vi "test Path Functions.vi"(8 "error in (no error)":errorcluster, 11 "TestCase in":refnum<class "Variant Data Manipulation Tests.lvclass">) -> (0 "error out":errorcluster, 3 "TestCase out":refnum<class "Variant Data Manipulation Tests.lvclass">)   [LabVIEW 2017, in "Variant Data Manipulation Tests.lvclass"]
uses:
  Variant Data Manipulation Tests.lvclass
  Source/Path API/Read Value at Path(String).vi
  Source/Path API/Write Value at Path(String).vi
  Source/Path API/Write Label at Path(String).vi
  <vilib>/addons/_JKI Toolkits/VI Tester/TestCase.llb/TestCase.lvclass
  Source/Variant Data Manipulation.lvlib
  C:/Program Files (x86)/National Instruments/LabVIEW 2017/vi.lib/addons/_JKI Toolkits/VI Tester/TestCase.llb/TestCase.lvclass
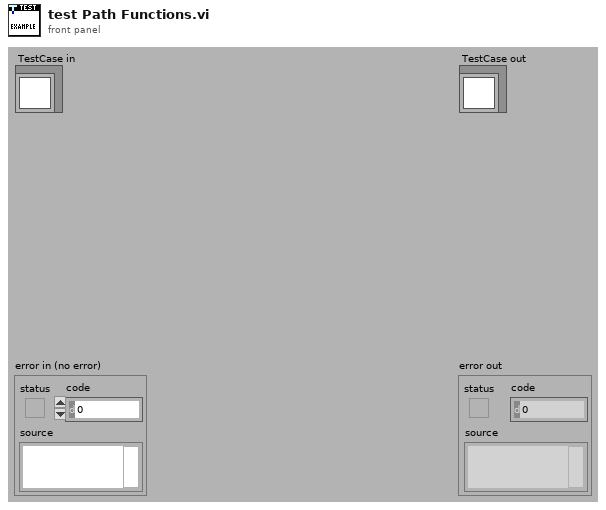
[diagram p1: front panel]
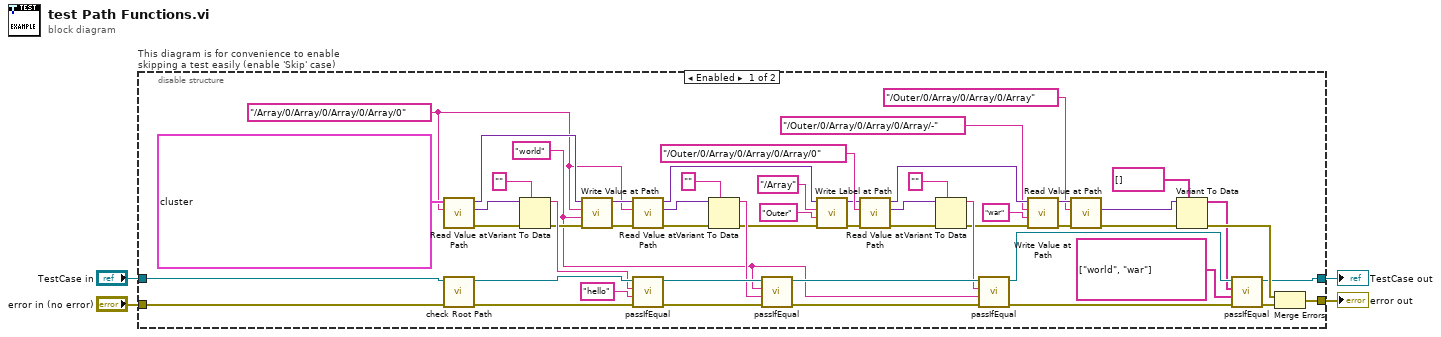
[diagram p0: block diagram]
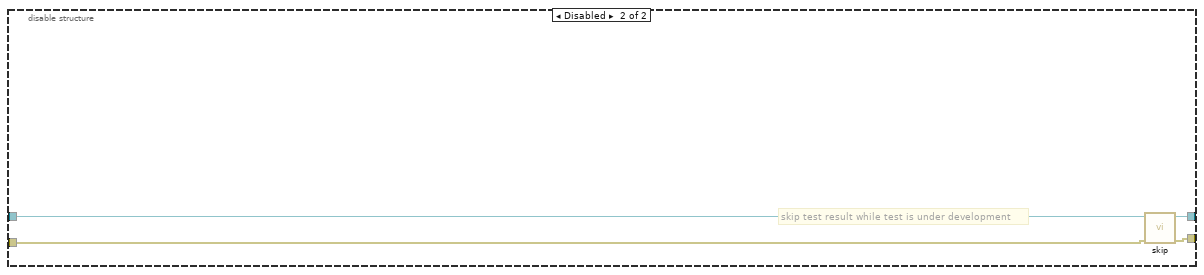
[diagram p2: hidden frame]
diagram:
  n1 = disable-structure "This diagram is for convenience to enable skipping a test easily (enable 'Skip' case)" shown="Enabled" {
    disable-tunnel: "TestCase in" -> [w57 w61]
    disable-tunnel: [w9 w59] -> w1
    disable-tunnel: [w24 w60] -> w3
    disable-tunnel: "error in (no error)" -> [w56 w58]
    frame Enabled {
      w21 = "world" ("String")
      w26 = "/Array/0/Array/0/Array/0/Array/0" ("Path String")
      n2 = call-poly "Read Value at Path.vi"("Path String"=w26, "Variant in"=cluster{"Array":cluster{"Array":cluster[]}[]} {"Array"=[{"Array"=[{"Array"=[{"Array"=["hello"]}]}]}]} ("Cluster")) -> ("error out"=w53:errorcluster, "Element out"=w52:variant, "Variant out"=w46:variant)  [unwired: 7 in]
      n3 = call "check Root Path.vi"("error in (no error)"=w56, "Variant Data Manipulation Tests in"=w57) -> ("error out"=w55:errorcluster, "Variant Data Manipulation Tests out"=w49:refnum<class "Variant Data Manipulation Tests.lvclass">)  [unwired: 8 in]
      n4 = Variant To Data(error in=w53, type="" ("String"), Variant=w52) -> (data=w48:string, error out=w41:errorcluster)
      n5 = call-poly "Write Value at Path.vi"("error in (no error)"=w41, "Element in"=w21, "Path String"=w26, "Variant in"=w46) -> ("error out"=w42:errorcluster, "Variant out"=w45:variant)  [unwired: 6 in]
      n6 = call-poly "Read Value at Path.vi"("error in (no error)"=w42, "Path String"=w26, "Variant in"=w45) -> ("error out"=w43:errorcluster, "Element out"=w37:variant, "Variant out"=w22:variant)  [unwired: 6 in]
      n7 = call-dynamic "passIfEqual.vi"("error in (no error)"=w55, "y"="hello" ("String"), "x"=w48, "TestCase in"=w49) -> ("error out"=w50:errorcluster, "TestCase out"=w39:refnum<class "Variant Data Manipulation Tests.lvclass">)  [unwired: 6 in]
      n8 = Variant To Data(error in=w43, type="" ("String"), Variant=w37) -> (data=w38:string, error out=w35:errorcluster)
      n9 = call-dynamic "passIfEqual.vi"("error in (no error)"=w50, "y"=w38, "x"=w21, "TestCase in"=w39) -> ("error out"=w40:errorcluster, "TestCase out"=w28:refnum<class "Variant Data Manipulation Tests.lvclass">)  [unwired: 6 in]
      n10 = call-poly "Write Label at Path.vi"("error in (no error)"=w35, "Name"="Outer", "Path String"="/Array" ("Path in"), "Variant in"=w22) -> ("error out"=w33:errorcluster, "Variant out"=w23:variant)  [unwired: 6 in]
      n11 = call-poly "Read Value at Path.vi"("error in (no error)"=w33, "Path String"="/Outer/0/Array/0/Array/0/Array/0", "Variant in"=w23) -> ("error out"=w25:errorcluster, "Element out"=w31:variant, "Variant out"=w20:variant)  [unwired: 6 in]
      n12 = Variant To Data(error in=w25, type="" ("String"), Variant=w31) -> (data=w27:string, error out=w14:errorcluster)
      n13 = call-dynamic "passIfEqual.vi"("error in (no error)"=w40, "y"=w21, "x"=w27, "TestCase in"=w28) -> ("error out"=w29:errorcluster, "TestCase out"=w10:refnum<class "Variant Data Manipulation Tests.lvclass">)  [unwired: 6 in]
      n14 = call-poly "Write Value at Path.vi"("error in (no error)"=w14, "Element in"="war" ("String"), "Path String"="/Outer/0/Array/0/Array/0/Array/-", "Variant in"=w20) -> ("error out"=w13:errorcluster, "Variant out"=w18:variant)  [unwired: 6 in]
      n15 = call-poly "Read Value at Path.vi"("error in (no error)"=w13, "Path String"="/Outer/0/Array/0/Array/0/Array", "Variant in"=w18) -> ("error out"=w16:errorcluster, "Element out"=w5:variant)  [unwired: 6 in, 1 out]
      n16 = Variant To Data(error in=w16, type=string[] [] ("String"), Variant=w5) -> (data=w8:string[], error out=w12:errorcluster)
      n17 = call-dynamic "passIfEqual.vi"("error in (no error)"=w29, "y"=string[] ["world", "war"] ("String"), "x"=w8, "TestCase in"=w10) -> ("error out"=w11:errorcluster, "TestCase out"=w9:refnum<class "Variant Data Manipulation Tests.lvclass">)  [unwired: 6 in]
      n18 = Merge Errors(w12, w11) -> (w24:errorcluster)
    }
    frame Disabled {
      # "skip test result while test is under development"
      n19 = call <vilib>:"skip.vi"("error in (no error)"=w58, "TestCase in"=w61) -> ("error out"=w60:errorcluster, "TestCase out"=w59:refnum<class "Variant Data Manipulation Tests.lvclass">)  [unwired: 8 in]
    }
  }
  "error out" <- w3
  "TestCase out" <- w1
